vi "sweep_mode_command.vi"(10 "Number of Sweeps":dbl, 11 "Sweep Mode":bool) -> (2 "Command Out":string)   [LabVIEW 2015]
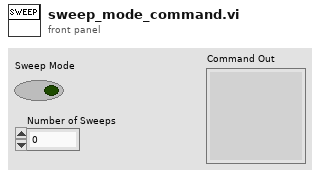
[diagram p1: front panel]
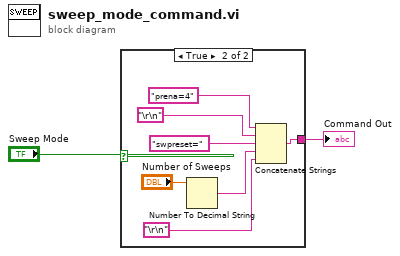
[diagram p0: block diagram]
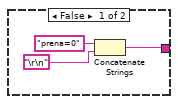
[diagram p2: hidden frame]
diagram:
  n1 = case shown="True" "Sweep Mode" {
    tunnel: [w5 w7] -> w1
    frame False {
      n2 = Concatenate Strings("prena=0" ("string"), "\r\n") -> (w5:string)
    }
    frame True {
      n3 = Number To Decimal String(number="Number of Sweeps") -> (decimal integer string=w8:string)  [unwired: 1 in]
      n4 = Concatenate Strings("prena=4", "\r\n", "swpreset=" ("string"), w8, "\r\n") -> (w7:string)
    }
  }
  "Command Out" <- w1
